vi "Create Range Array.vi"(9 "Delta":dbl, 10 "To":dbl, 11 "From":dbl) -> (3 "Array":dbl[](array[numeric]))   [LabVIEW 2014, in "SimpleExperimentService.lvclass"]
uses:
  SimpleExperimentService.lvclass
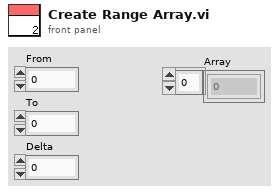
[diagram p1: front panel]
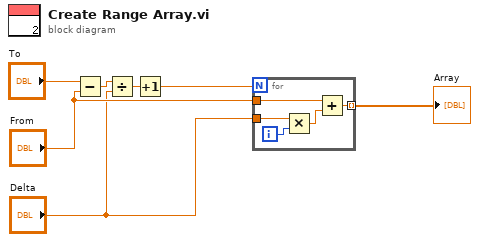
[diagram p0: block diagram]
diagram:
  n1 = Subtract(x="To", y="From") -> (x-y=w2:dbl)
  n2 = Divide(x=w2, y="Delta") -> (x/y=w5:dbl)
  n3 = Increment(x=w5) -> (x+1=w6:dbl)
  n4 = for {
    N: w6 -> [_]
    tunnel: "Delta" -> [w11]
    tunnel: "From" -> [w9]
    tunnel: [w8] -> w7 mode=indexing
    i -> [w12]
    n5 = Multiply(x=w11, y=w12) -> (x*y=w10:dbl)
    n6 = Add(x=w9, y=w10) -> (x+y=w8:dbl)
  }
  "Array" <- w7
